vi "plotToLongDAQ.vi"(8 "DAQ3":refnum<vi>, 9 "DAQ2":refnum<vi>, 10 "DAQ1":refnum<vi>, 11 "Experiment State":T1={"error"={"status"=FALSE, "code"=0, "source"=""}, "Digitizer DAQmx Tasks"={"TaskArray"=[]}, "Digitizer Settings"={"Channel Settings"=[], "Card Settings"=[]}, "Synchronization Settings"={"Synchronizer"="PXI1Slot2", "source terminal"="GlobalSoftwareTrigger"}, "Digitizer Data"=[], "Next Shot#"="0", "System Message"="", "User Shot Notes"="", "Timing Settings"={"Timing Card Settings"=[], "Timing Channel Settings"=[[{"Delay (s)"=2.559999942779541, "Pulse width (s)"=0.009999999776482582, "Active"=TRUE, "Channel Name"="Fiber 8", "counter"="PXI1Slot8/ctr7"}]]}, "Timing Tasks"={"TaskArray"=[]}} {"Timing Settings"."Timing Channel Settings"."Pulse width (s)" format="%.3p"; "Timing Settings"."Timing Channel Settings"."Delay (s)" format="%.3p"; "Digitizer Settings"."Card Settings"."Global Edge Type" items=["Rising"=10280, "Falling"=10171]; "Digitizer Settings"."Card Settings"."Sample Rate" format="%#_3p"}) -> ()   [LabVIEW 2013]
uses:
  Controls/ExperimentStateCluster.ctl
  Controls/DigitizerSettingsChannelSettings.ctl
  Controls/DigitizerSettingsCardSettingsArray.ctl
  Controls/DigitizerSettingsCardSettings.ctl
  Controls/TimingCardSettings.ctl
  Controls/TimingChannelSettings.ctl
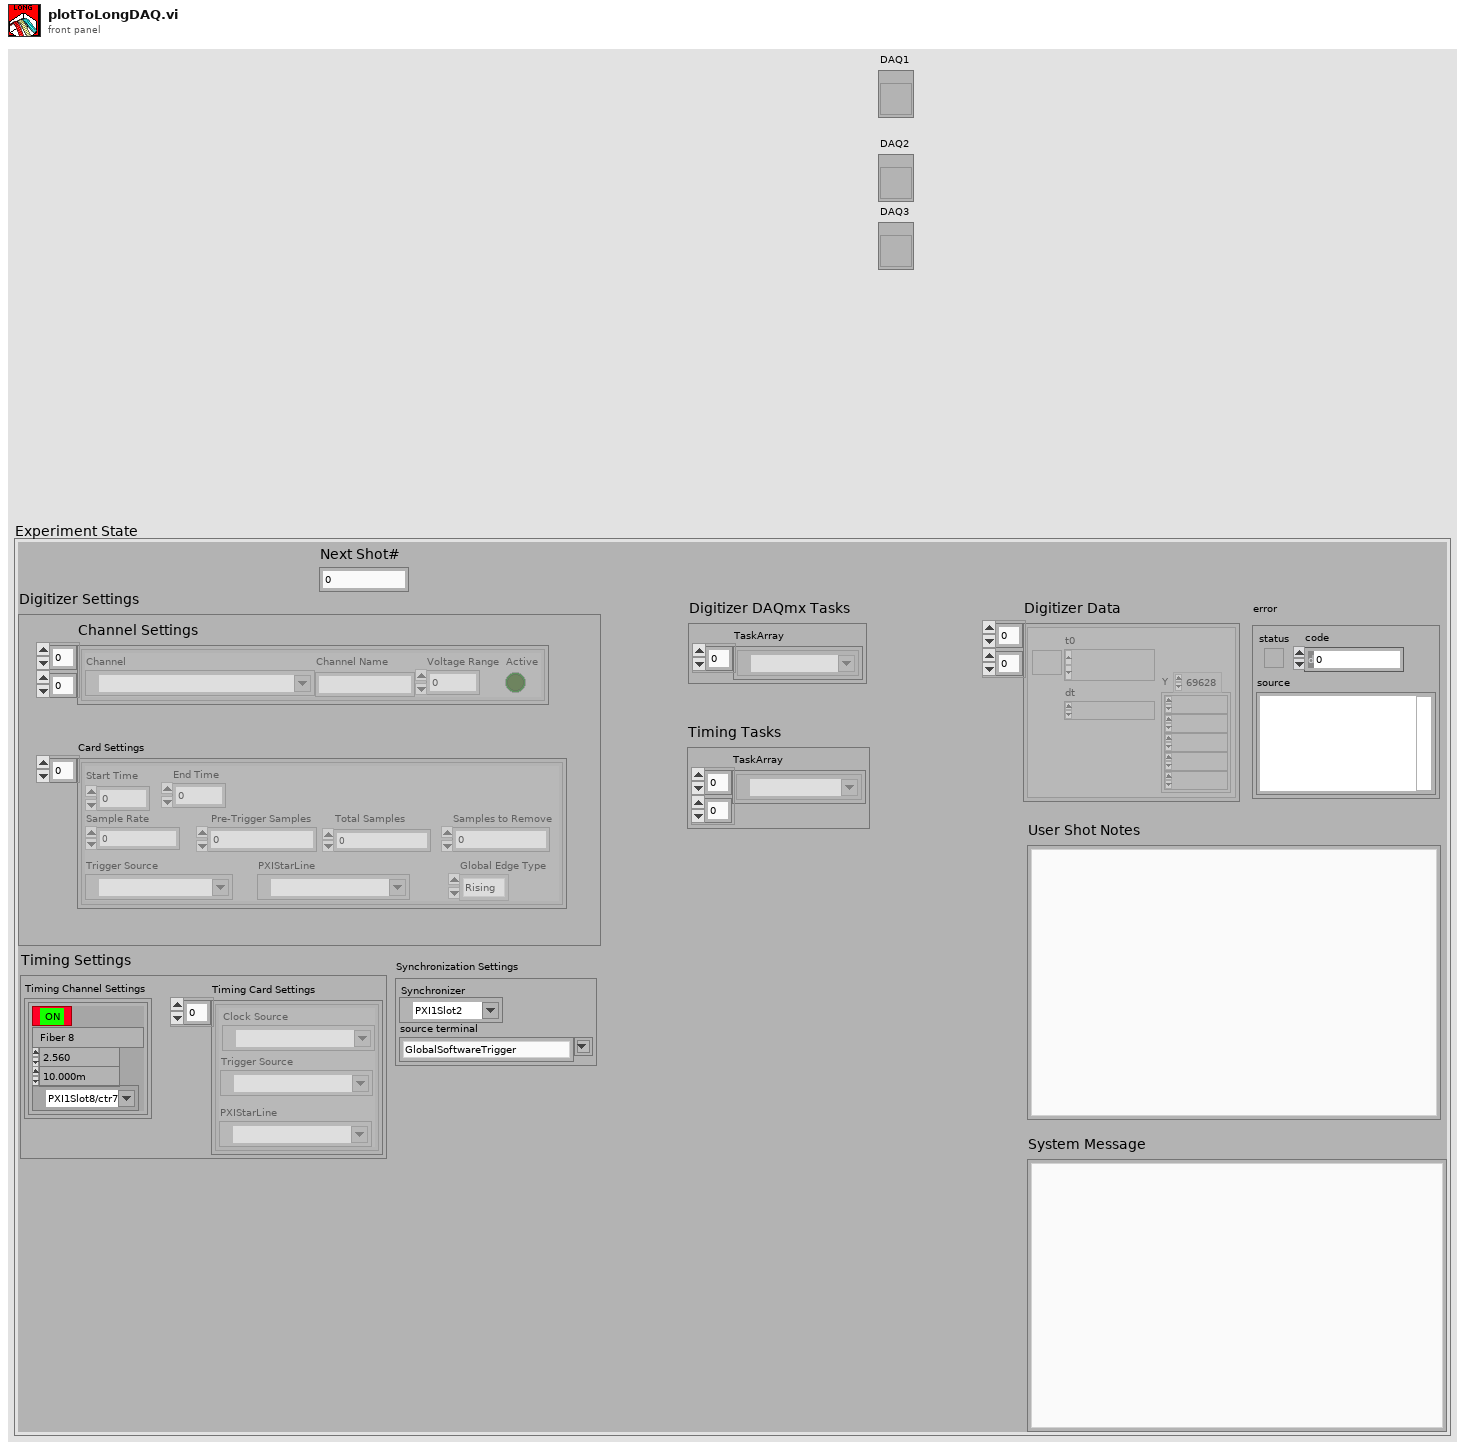
[diagram p1: front panel]
types:
  T1 = typedef "ExperimentStateCluster.ctl" = cluster{"error":errorcluster, "Digitizer DAQmx Tasks":cluster{"TaskArray":refnum<k21>[]}, "Digitizer Settings":cluster{"Channel Settings":T2[][], "Card Settings":T3}, "Synchronization Settings":cluster{"Synchronizer":refnum<k15>, "source terminal":string}, "Digitizer Data":waveform(dbl)[][], "Next Shot#":string, "System Message":string, "User Shot Notes":string, "Timing Settings":cluster{"Timing Card Settings":T5[], "Timing Channel Settings":T6[][]}, "Timing Tasks":cluster{"TaskArray":refnum<k21>[][]}}
  T2 = typedef "DigitizerSettingsChannelSettings.ctl" = cluster{"Channel":tag, "Channel Name":string, "Voltage Range":dbl, "Active":bool}
  T3 = typedef "DigitizerSettingsCardSettingsArray.ctl" = T4[]
  T4 = typedef "DigitizerSettingsCardSettings.ctl" = cluster{"Start Time":dbl, "End Time":dbl, "Sample Rate":dbl, " Pre-Trigger Samples":u32, "Total Samples":i32, "Samples to Remove":u32, "Trigger Source":tag, "Global Edge Type":i32, "PXIStarLine":tag}
  T5 = typedef "TimingCardSettings.ctl" = cluster{"Trigger Source":tag, "Clock Source":tag, "PXIStarLine":tag}
  T6 = typedef "TimingChannelSettings.ctl" = cluster{"Delay (s)":dbl, "Pulse width (s)":dbl, "Active":bool, "Channel Name":string, "counter":tag}
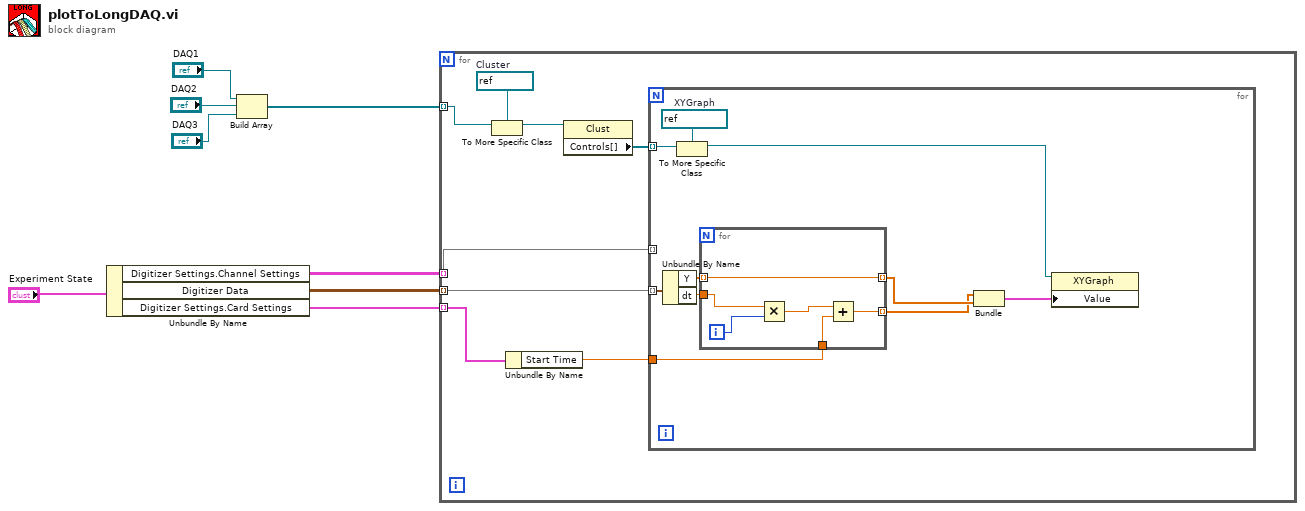
[diagram p0: block diagram]
diagram:
  n1 = Unbundle By Name("Experiment State") -> ("Digitizer Settings.Channel Settings"=w1:T2[][], "Digitizer Data"=w4:waveform(dbl)[][], "Digitizer Settings.Card Settings"=w2:T3)
  n2 = Build Array("DAQ1", "DAQ2", "DAQ3") -> (w3:refnum<vi>[])
  n3 = for {
    tunnel: w4 -> [w13] mode=indexing
    tunnel: w3 -> [w16] mode=indexing
    tunnel: w2 -> [w11] mode=indexing
    tunnel: w1 -> [w9] mode=indexing
    w15 = refnum<vi> refnum  # Cluster
    n4 = To More Specific Class(target class=w15, reference=w16) -> (specific class reference=w14:refnum<vi>)  [unwired: 1 in, 1 out]
    n5 = Unbundle By Name(w11) -> ("Start Time"=w10:dbl)
    n6 = property class="Clust"(reference=w14) -> ("Controls[]"=w12:refnum<vi>[])  [unwired: 1 in, 2 out]
    n7 = for {
      tunnel: w13 -> [w24] mode=indexing
      tunnel: w12 -> [w26] mode=indexing
      tunnel: w10 -> [w17]
      tunnel: w9 -> [_] mode=indexing
      w25 = refnum<vi> refnum  # XYGraph
      n8 = Unbundle By Name(w24) -> ("Y"=w23:dbl[], "dt"=w22:dbl)
      n9 = To More Specific Class(target class=w25, reference=w26) -> (specific class reference=w18:refnum<vi>)  [unwired: 1 in, 1 out]
      n10 = for {
        tunnel: w23 -> [w32] mode=indexing
        tunnel: w22 -> [w31]
        tunnel: [w32] -> w21 mode=indexing
        tunnel: [w27] -> w20 mode=indexing
        tunnel: w17 -> [w29]
        i -> [w30]
        n11 = Multiply(x=w31, y=w30) -> (x*y=w28:dbl)
        n12 = Add(x=w28, y=w29) -> (x+y=w27:dbl)
      }
      n13 = Bundle(w20, w21) -> (w19:cluster{dbl[], dbl[]})  [unwired: 1 in]
      n14 = property class="XYGraph"(reference=w18, "Value"=w19) -> ()  [unwired: 1 in, 2 out]
    }
  }
